vi "AverageTempF.vi"(11 "Array":string[](array[string])) -> (3 "Boolean":bool)   [LabVIEW 2015]
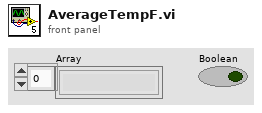
[diagram p1: front panel]
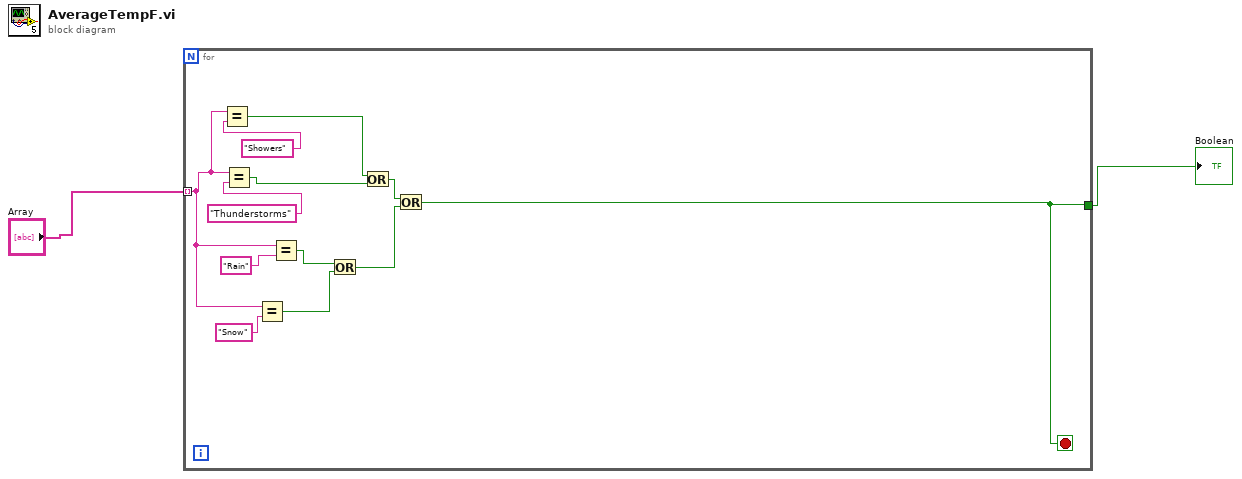
[diagram p0: block diagram]
diagram:
  n1 = for {
    tunnel: "Array" -> [w7] mode=indexing
    tunnel: [w3] -> w2
    stop <- w3 stop-if-true
    n2 = Equal?(x=w7, y="Showers") -> (x = y?=w11:bool)
    n3 = Equal?(x=w7, y="Thunderstorms") -> (x = y?=w10:bool)
    n4 = Equal?(x=w7, y="Snow") -> (x = y?=w5:bool)
    n5 = Equal?(x=w7, y="Rain") -> (x = y?=w6:bool)
    n6 = Or(x=w6, y=w5) -> (x .or. y?=w4:bool)
    n7 = Or(x=w11, y=w10) -> (x .or. y?=w9:bool)
    n8 = Or(x=w9, y=w4) -> (x .or. y?=w3:bool)
  }
  "Boolean" <- w2
